vi "Init RC Servo.vi"(8 "error in (no error)":errorcluster, 10 "GPIO":i32, 11 "VISA resource name in":refnum<visa-resource-name>) -> (0 "error out":errorcluster, 3 "VISA resource name":refnum<visa-resource-name>)   [LabVIEW 2023, in "CTI-Visa.lvlib"]
uses:
  CTI-Visa.lvlib
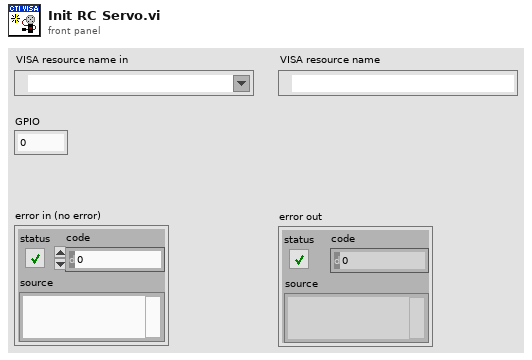
[diagram p1: front panel]
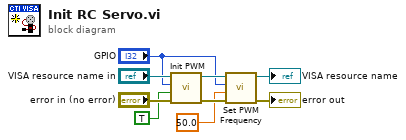
[diagram p0: block diagram]
diagram:
  n1 = call "Init PWM.vi"("error in (no error)"="error in (no error)", "Enable (F)"=TRUE, "Channel"="GPIO", "VISA resource name in"="VISA resource name in") -> ("error out"=w9:errorcluster, "VISA resource name"=w6:refnum<visa-resource-name>)  [unwired: 6 in]
  n2 = call "Set PWM Frequency.vi"("error in (no error)"=w9, "Freq Hz"=sgl 50.0, "Channel"="GPIO", "VISA resource name in"=w6) -> ("error out"=→"error out":errorcluster, "VISA resource name"=→"VISA resource name":refnum<visa-resource-name>)  [unwired: 6 in]
